vi "StorePAQ_10mil.vi"(8 "error in (no error)":errorcluster, 10 "StoreDatagram":T1 {"Time" format="%#.2f"; "status" format="%x"; "min" format="%.2f"; "max" format="%.2f"; "data" format="%.2f"}, 11 "FAMM in":refnum<class "FAMM.lvclass">) -> (0 "error out":errorcluster, 3 "FAMM out":refnum<class "FAMM.lvclass">)   [LabVIEW 2014, in "FAMM.lvclass"]
doc: "Store one element to the 10 millisecond memory"
uses:
  FAMM.lvclass
  controls/MemStoreDatagram.ctl
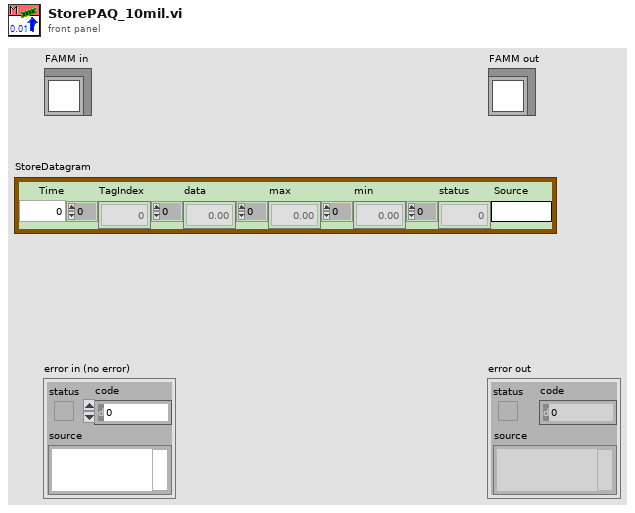
[diagram p1: front panel]
types:
  T1 = typedef "MemStoreDatagram.ctl" = cluster{"Time":dbl, "TagIndex":i32[], "data":dbl[], "max":dbl[], "min":dbl[], "status":u32[], "Source":string}
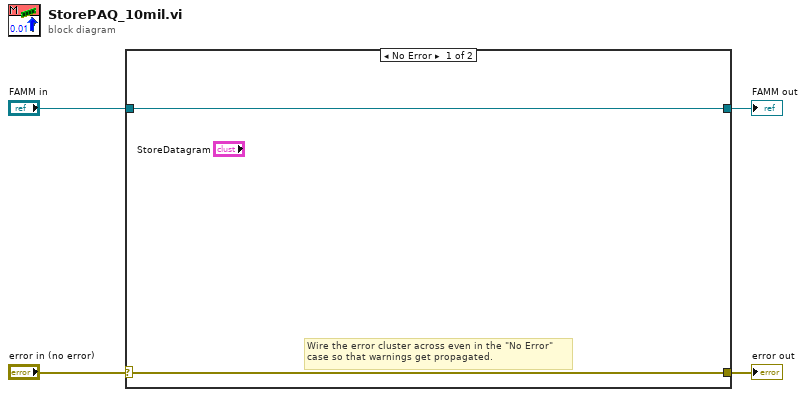
[diagram p0: block diagram]
diagram:
  n1 = case shown="No Error" "error in (no error)" {
    selector: "error in (no error)" -> [w5 w8]
    tunnel: [w5 w8] -> w3
    tunnel: [w6 w7] -> w1
    tunnel: "FAMM in" -> [w6 w7]
    frame No Error {
      # "Wire the error cluster across even in the \"No Error\"\ncase so that warnings get propagated."
    }
    frame Error {
    }
  }
  "error out" <- w3
  "FAMM out" <- w1
